vi "SET_Text.vi"(8 "error in (no error)":errorcluster, 10 "Text":T1={"Font"="", "Alignment"=enum."left", "Size"=3} {"Size" min=3 max=32 step=1}, 11 "Settings.lvclass in":refnum<class "Settings.lvclass">) -> (0 "error out":errorcluster, 3 "Settings.lvclass out":refnum<class "Settings.lvclass">)   [LabVIEW 2020, in "Settings.lvclass"]
uses:
  Settings.lvclass
  Settings.lvclass/Settings.ctl
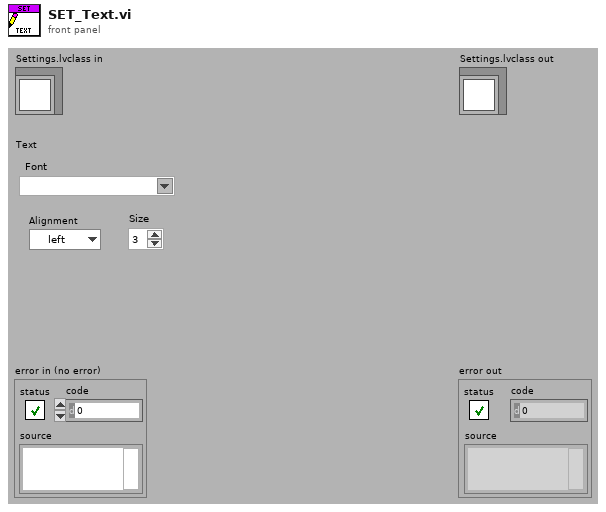
[diagram p1: front panel]
types:
  T1 = cluster{"Font":string, "Alignment":enum16{"left", "center", "right"}, "Size":u8}
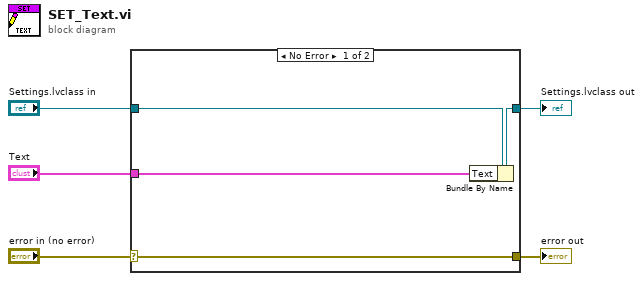
[diagram p0: block diagram]
diagram:
  n1 = case shown="No Error" "error in (no error)" {
    selector: "error in (no error)" -> [w9 w10]
    tunnel: [w9 w10] -> w4
    tunnel: [w7 w11] -> w2
    tunnel: "Settings.lvclass in" -> [w8 w11]
    tunnel: "Text" -> [w6 _]
    frame No Error {
      n2 = Bundle By Name(cluster=w8, "Text"=w6) -> (w7:refnum<class "Settings.lvclass">)
    }
    frame Error {
    }
  }
  "error out" <- w4
  "Settings.lvclass out" <- w2
